vi "Is Valid.vi"(8 "error in (no error)":errorcluster, 11 "Result in":refnum<class "Task.lvclass">) -> (0 "error out":errorcluster, 2 "Valid":bool, 3 "Result out":refnum<class "Task.lvclass">)   [LabVIEW 2017, in "Futures.lvlib" / "Task.lvclass"]
uses:
  Task.lvclass
  Task.lvclass/Task.ctl
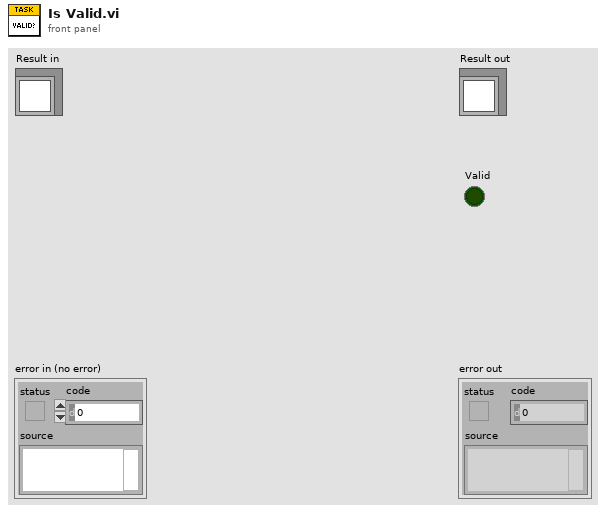
[diagram p1: front panel]
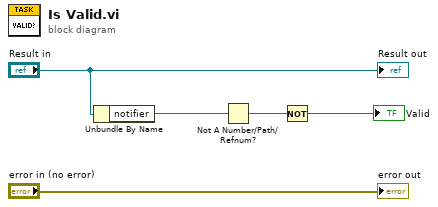
[diagram p0: block diagram]
diagram:
  n1 = Unbundle By Name("Result in") -> ("notifier"=w2:refnum<notifier>)
  n2 = Not A Number/Path/Refnum?(number/path/refnum=w2) -> (NaN/Path/Refnum?=w1:bool)
  n3 = Not(x=w1) -> (.not. x?=→"Valid":bool)
  "error out" <- "error in (no error)"
  "Result out" <- "Result in"
